vi "CIF Channels Post-Install Custom Action.vi"(10 "Variant":variant) -> (0 "error out":errorcluster)   [LabVIEW 2021]
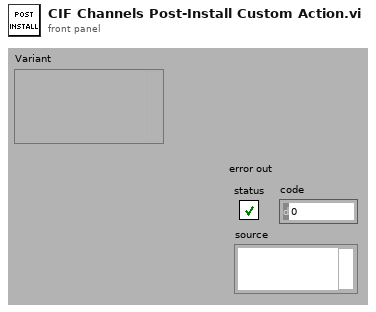
[diagram p1: front panel]
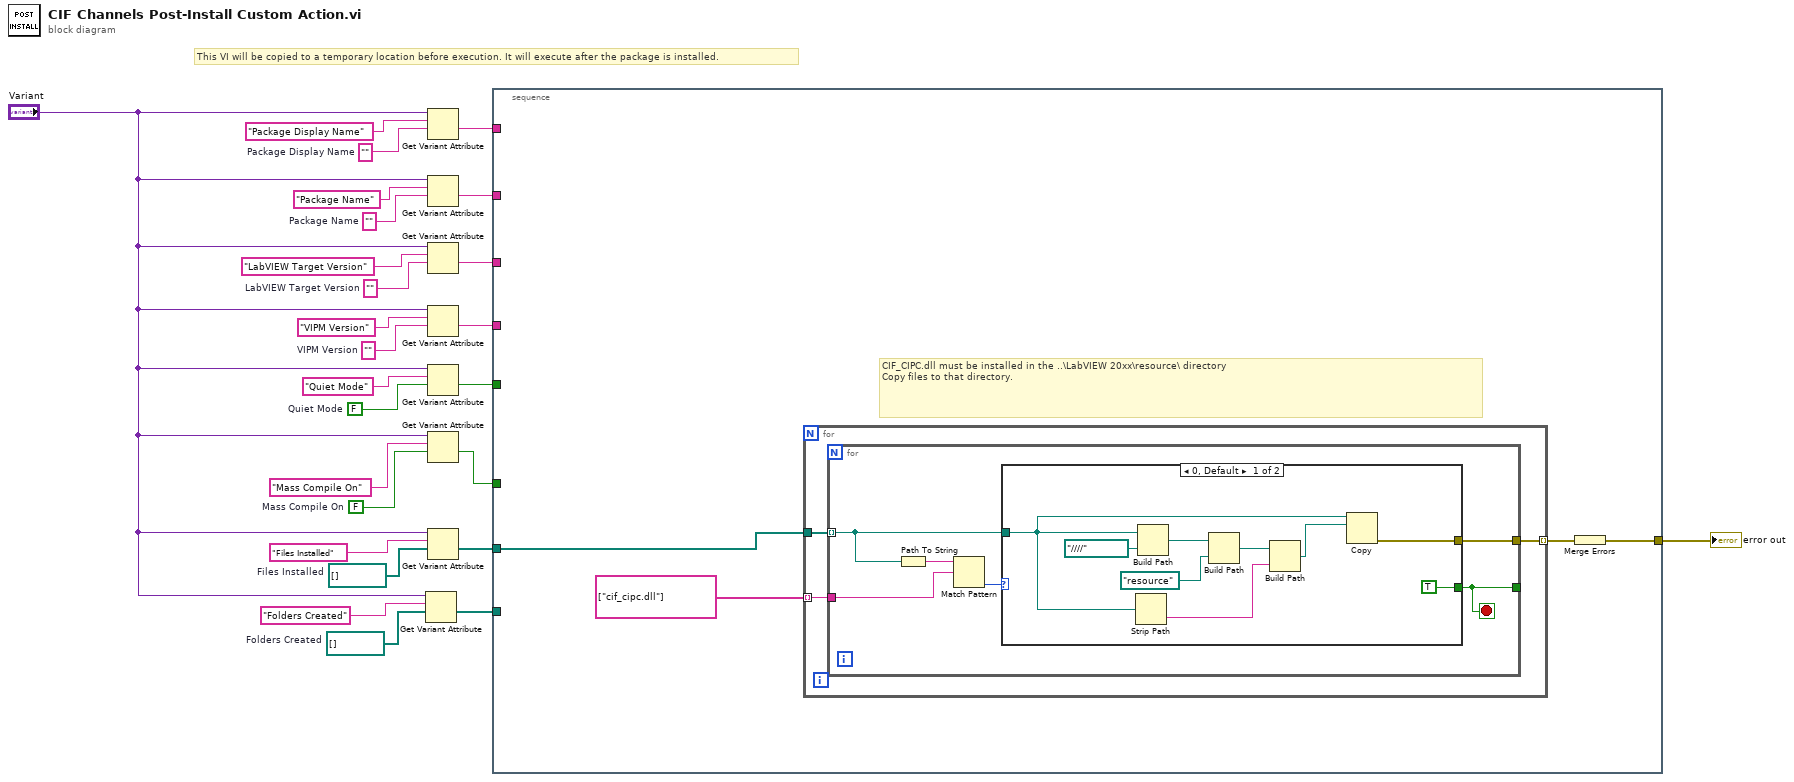
[diagram p0: block diagram]
diagram:
  w2 = path[] []  # Folders Created
  w3 = path[] []  # Files Installed
  w9 = FALSE  # Mass Compile On
  w10 = ""  # Package Display Name
  w17 = FALSE  # Quiet Mode
  w20 = ""  # VIPM Version
  w22 = ""  # LabVIEW Target Version
  w24 = ""  # Package Name
  # "This VI will be copied to a temporary location before execution. It will execute after the package is installed."
  n1 = Get Variant Attribute(Variant="Variant", name="Folders Created", default value (empty Variant)=w2) -> (value=w7:path[])  [unwired: 1 in, 3 out]
  n2 = Get Variant Attribute(Variant="Variant", name="Package Display Name", default value (empty Variant)=w10) -> (value=w16:string)  [unwired: 1 in, 3 out]
  n3 = Get Variant Attribute(Variant="Variant", name="Package Name", default value (empty Variant)=w24) -> (value=w15:string)  [unwired: 1 in, 3 out]
  n4 = Get Variant Attribute(Variant="Variant", name="LabVIEW Target Version", default value (empty Variant)=w22) -> (value=w14:string)  [unwired: 1 in, 3 out]
  n5 = Get Variant Attribute(Variant="Variant", name="VIPM Version", default value (empty Variant)=w20) -> (value=w13:string)  [unwired: 1 in, 3 out]
  n6 = Get Variant Attribute(Variant="Variant", name="Quiet Mode", default value (empty Variant)=w17) -> (value=w12:bool)  [unwired: 1 in, 3 out]
  n7 = Get Variant Attribute(Variant="Variant", name="Mass Compile On", default value (empty Variant)=w9) -> (value=w11:bool)  [unwired: 1 in, 3 out]
  n8 = Get Variant Attribute(Variant="Variant", name="Files Installed", default value (empty Variant)=w3) -> (value=w6:path[])  [unwired: 1 in, 3 out]
  n9 = stacked-sequence {
    tunnel: w16 -> [_]
    tunnel: w15 -> [_]
    tunnel: w14 -> [_]
    tunnel: w13 -> [_]
    tunnel: w12 -> [_]
    tunnel: w11 -> [_]
    tunnel: w6 -> [w29]
    tunnel: w7 -> [_]
    tunnel: [w27] -> w1
    frame #0 {
      # "CIF_CIPC.dll must be installed in the ..\\LabVIEW 20xx\\resource\\ directory\nCopy files to that directory."
      n10 = for {
        tunnel: w29 -> [w33]
        tunnel: string[] ["cif_cipc.dll"] -> [w32] mode=indexing
        tunnel: [w31] -> w28 mode=indexing
        n11 = for {
          tunnel: w33 -> [w37] mode=indexing
          tunnel: [w36] -> _
          tunnel: w32 -> [w35]
          tunnel: [w34] -> w31
          stop <- w36 stop-if-true
          n12 = Path To String(path=w37) -> (string=w39:string)
          n13 = Match Pattern(string=w39, regular expression=w35) -> (offset past match=w38:i32)  [unwired: 1 in, 3 out]
          n14 = case shown="0, Default" w38 {
            tunnel: w37 -> [w41 _]
            tunnel: [TRUE _] -> w36
            tunnel: [w40 _] -> w34
            frame 0, Default {
              n15 = Strip Path(path=w41) -> (name=w44:string)  [unwired: 1 out]
              n16 = Build Path(base path=w41, name or relative path=path "../../../../..") -> (appended path=w47:path)
              n17 = Build Path(base path=w47, name or relative path=path "resource") -> (appended path=w45:path)
              n18 = Build Path(base path=w45, name or relative path=w44) -> (appended path=w42:path)
              n19 = Copy(10:w42, 11:w41) -> (0:w40:errorcluster)  [unwired: 3 in, 2 out]
            }
            frame -1 {
            }
          }
        }
      }
      n20 = Merge Errors(w28) -> (w27:errorcluster)
    }
  }
  "error out" <- w1
